vi "copy constants from config.vi"(8 "error in (no error)":errorcluster, 10 "PID Loops":refnum<class "PID Loop.lvclass">[](array[class]), 11 "Tagbus PID Module runtime in":refnum<class "PID Module runtime.lvclass">) -> (0 "error out":errorcluster, 3 "Tagbus PID Module runtime out":refnum<class "PID Module runtime.lvclass">)   [LabVIEW 2013, in "PID Module runtime.lvclass"]
uses:
  PID Module runtime.lvclass
  configuration/PID Loop.lvclass
  PID Module runtime.lvclass/PID Module runtime.ctl
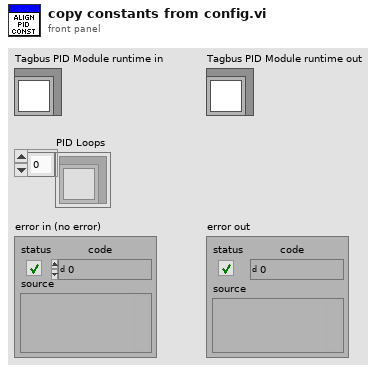
[diagram p1: front panel]
types:
  T1 = typedef "PID Loop.lvclass/PID Gains.ctl" = cluster{"proportional gain (Kc)":dbl, "integral time (Ti, min)":dbl, "derivative time (Td, min)":dbl}
  T2 = typedef "PID Loop.lvclass/PID Range.ctl" = cluster{"output high":dbl, "output low":dbl}
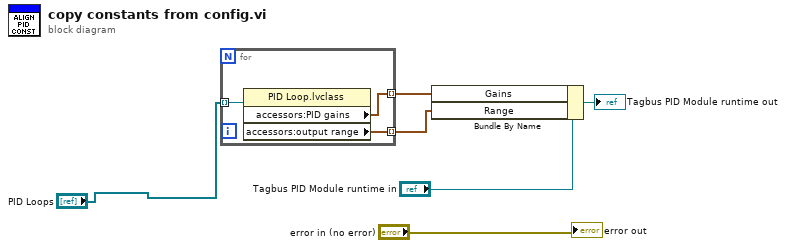
[diagram p0: block diagram]
diagram:
  n1 = for {
    tunnel: "PID Loops" -> [w9] mode=indexing
    tunnel: [w8] -> w2 mode=indexing
    tunnel: [w7] -> w1 mode=indexing
    n2 = property class="PID Loop.lvclass"(reference=w9) -> ("accessors:PID gains"=w8:T1, "accessors:output range"=w7:T2)  [unwired: 1 in, 2 out]
  }
  n3 = Bundle By Name(cluster="Tagbus PID Module runtime in", "Gains"=w2, "Range"=w1) -> (→"Tagbus PID Module runtime out":refnum<class "PID Module runtime.lvclass">)
  "error out" <- "error in (no error)"
